vi "to string 2.0.vi"(8 "error in":errorcluster, 10 "data in":string, 11 "Shared Memory configuration in":refnum<class "Shared Memory configuration.lvclass">) -> (0 "error out":errorcluster, 2 "data out":string, 3 "Shared Memory configuration out":refnum<class "Shared Memory configuration.lvclass">)   [LabVIEW 2013, in "Shared Memory configuration.lvclass"]
uses:
  Shared Memory configuration.lvclass
  Shared Memory configuration.lvclass/Shared Memory configuration.ctl
  <vilib>/NI/Tag Bus Module Framework/channel/TBM channel.lvclass
  <vilib>/NI/Configuration Framework/serializable configuration/NISE_CEF_serializable configuration.lvclass
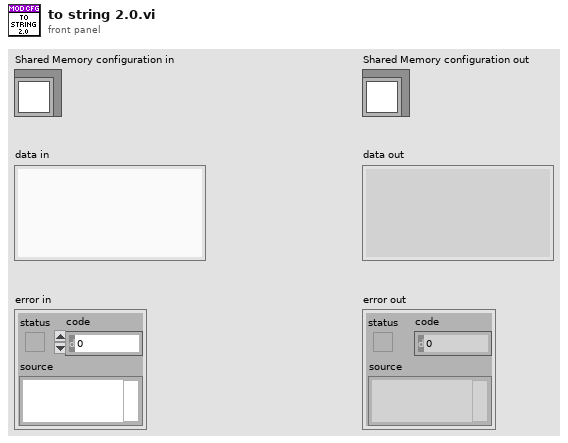
[diagram p1: front panel]
types:
  T1 = typedef "Shared Memory configuration.lvclass/Line.ctl" = cluster{"channel":refnum<class "TBM channel.lvclass">}
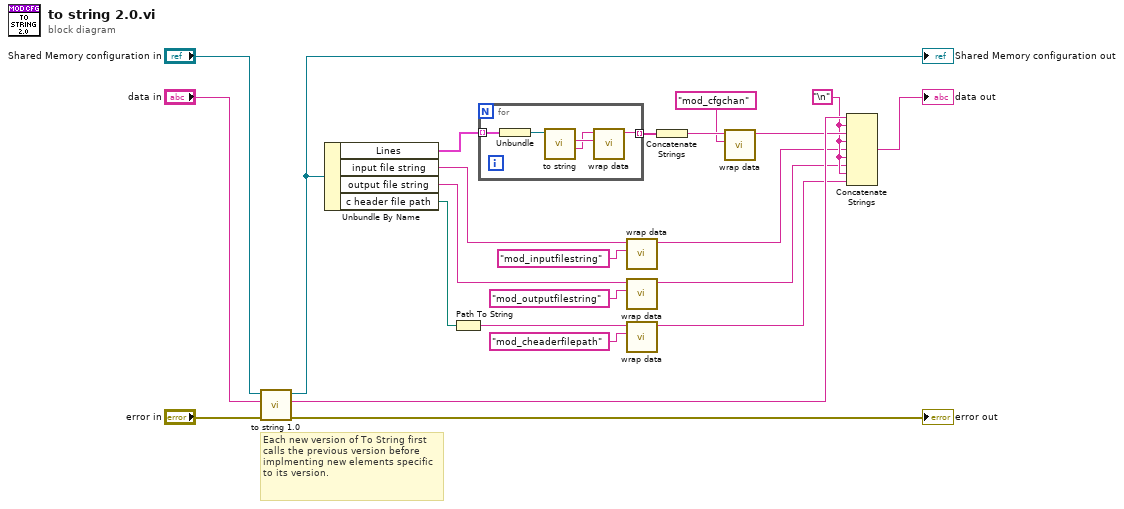
[diagram p0: block diagram]
diagram:
  w4 = "\n"
  # "Each new version of To String first calls the previous version before implmenting new elements specific to its version."
  n1 = call "to string 1.0.vi"("error in"="error in", "data in"="data in", "Shared Memory configuration in"="Shared Memory configuration in") -> ("error out"=→"error out":errorcluster, "data out"=w21:string, "Shared Memory configuration out"=w18:refnum<class "Shared Memory configuration.lvclass">)  [unwired: 6 in]
  "Shared Memory configuration out" <- w18
  n2 = Unbundle By Name(w18) -> ("Lines"=w13:T1[], "input file string"=w5:string, "output file string"=w6:string, "c header file path"=w7:path)
  n3 = Path To String(path=w7) -> (string=w8:string)
  n4 = for {
    tunnel: w13 -> [w28] mode=indexing
    tunnel: [w24] -> w16 mode=indexing
    n5 = Unbundle(w28) -> ("channel"=w27:refnum<class "TBM channel.lvclass">)
    n6 = call-dynamic "to string.vi"("channel in"=w27) -> ("channel data"=w25:string, "identifier"=w26:string)  [unwired: 7 in, 2 out]
    n7 = call <vilib>:"wrap data.vi"("identifier"=w26, "data to wrap"=w25) -> ("wrapped data"=w24:string)  [unwired: 9 in]
  }
  n8 = call <vilib>:"wrap data.vi"("identifier"="mod_inputfilestring", "data to wrap"=w5) -> ("wrapped data"=w3:string)  [unwired: 9 in]
  n9 = call <vilib>:"wrap data.vi"("identifier"="mod_outputfilestring", "data to wrap"=w6) -> ("wrapped data"=w2:string)  [unwired: 9 in]
  n10 = call <vilib>:"wrap data.vi"("identifier"="mod_cheaderfilepath", "data to wrap"=w8) -> ("wrapped data"=w1:string)  [unwired: 9 in]
  n11 = Concatenate Strings(w16) -> (w15:string)
  n12 = call <vilib>:"wrap data.vi"("identifier"="mod_cfgchan", "data to wrap"=w15) -> ("wrapped data"=w12:string)  [unwired: 9 in]
  n13 = Concatenate Strings(w21, w4, w12, w4, w3, w4, w2, w4, w1) -> (→"data out":string)
